vi "UpdateNavxData.vi"(9 "Iterations between saves":i32=10, 10 "Iteration counter":i32, 11 "Datalogging File Refnum in":refnum<k34>) -> (3 "Datalogging File Refnum out":refnum<k34>)   [LabVIEW 2014]
uses:
  Navx_Library/navX-MXP Library/COMMON/TypeDefs/Data TypeDefs/navX Quaternion Data.ctl
  Navx_Library/navX-MXP Library/COMMON/TypeDefs/Data TypeDefs/navX YPRH Data.ctl
  Navx_Library/navX-MXP Library/COMMON/TypeDefs/Data TypeDefs/navX Vector Data.ctl
  Variables/Physical data.vi
  Variables/Default global.vi
  Navx_Library/navX-MXP Library/navX-MXP IMU.lvlib
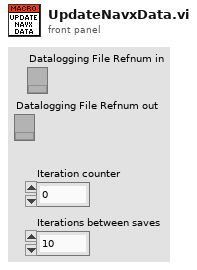
[diagram p1: front panel]
types:
  T1 = typedef "navX-MXP IMU.lvlib/navX Quaternion Data.ctl" = cluster{"W":dbl, "X":dbl, "Y":dbl, "Z":dbl}
  T2 = typedef "navX-MXP IMU.lvlib/navX YPRH Data.ctl" = cluster{"Yaw":dbl, "Pitch":dbl, "Roll":dbl, "Heading":dbl}
  T3 = typedef "navX-MXP IMU.lvlib/navX Vector Data.ctl" = cluster{"X":dbl, "Y":dbl, "Z":dbl}
  T4 = cluster{"Quaternion":T1, "YPRH":T2, "Linear Acceleration":T3, "Valid?":bool}
  T5 = typedef "navX-MXP IMU.lvlib/navX Device TypeDef.ctl" = cluster{"navX Interface Protocol":T6, "navX Interface Protocol TypeDefs":cluster{"SPIDevRef":T7, "I2CDevRef":T10}, "navX System Information":cluster{"Board Information":T12, "Status":T13, "Offsets":T17}, "navX Common Information":cluster{"Update Rate (4Hz-60Hz)":T18, "refnum name":string, "error":errorcluster}}
  T6 = typedef "navX-MXP IMU.lvlib/navX Interface Protocol.ctl" = enum16{"SPI", "I2C"}
  T7 = typedef "WPI_SPIDevRef.ctl" = cluster{"DevStatus":errorcluster, "Handle":i32, "Controller":T8, "SPI Bus":T9}
  T8 = typedef "FPGA_TypedefDigitalModule.ctl" = enum16{"Controller 1"}
  T9 = typedef "spi_bus.ctl" = enum16{"SPI On-Board, CS0", "SPI On-Board, CS1", "SPI On-Board, CS2", "SPI On-Board, CS3", "SPI MXP", "Invalid"}
  T10 = typedef "WPI_I2CDevRef.ctl" = cluster{"DevStatus":errorcluster, "Controller":T8, "Device Address":u8, "Handle":i32, "I2C Bus":T11}
  T11 = typedef "i2c_bus.ctl" = enum16{"I2C On-Board", "I2C MXP", "Invalid"}
  T12 = typedef "navX-MXP IMU.lvlib/navX Board Information.ctl" = cluster{"WhoAmI (50 | 0x32)":u8, "Board Revision":u8, "Firmware Major Version":u8, "Firmware Minor Version":u8}
  T13 = typedef "navX-MXP IMU.lvlib/navX Status Data.ctl" = cluster{"Update Rate Hz":u8, "Accelerometer Full-Scale Range":u8, "Gyro Full-Scale Range":u16, "NAVX_OP_STATUS":T14, "NAVX_CAL_STATUS":T15, "NAVX_SELFTEST_STATUS":u8, "NAVX_SENSOR_STATUS":T16}
  T14 = typedef "navX-MXP IMU.lvlib/navX NAVX_OP_STATUS.ctl" = u8
  T15 = typedef "navX-MXP IMU.lvlib/navX NAVX_CAL_STATUS.ctl" = u8
  T16 = typedef "navX-MXP IMU.lvlib/navX NAVX_SENSOR_STATUS.ctl" = cluster{"MOVING":bool, "YAW_STABLE":bool, "MAG_DISTURBANCE":bool, "ALTITUDE_VALID":bool, "SEALEVEL_PRESS_SET":bool, "FUSED_HEADING_VALID":bool}
  T17 = typedef "navX-MXP IMU.lvlib/navX Offsets Data.ctl" = cluster{"Yaw":dbl, "Quat W":dbl, "Quat X":dbl, "Quat Y":dbl, "Quat Z":dbl}
  T18 = typedef "navX-MXP IMU.lvlib/navX Update Rate.ctl" = u8
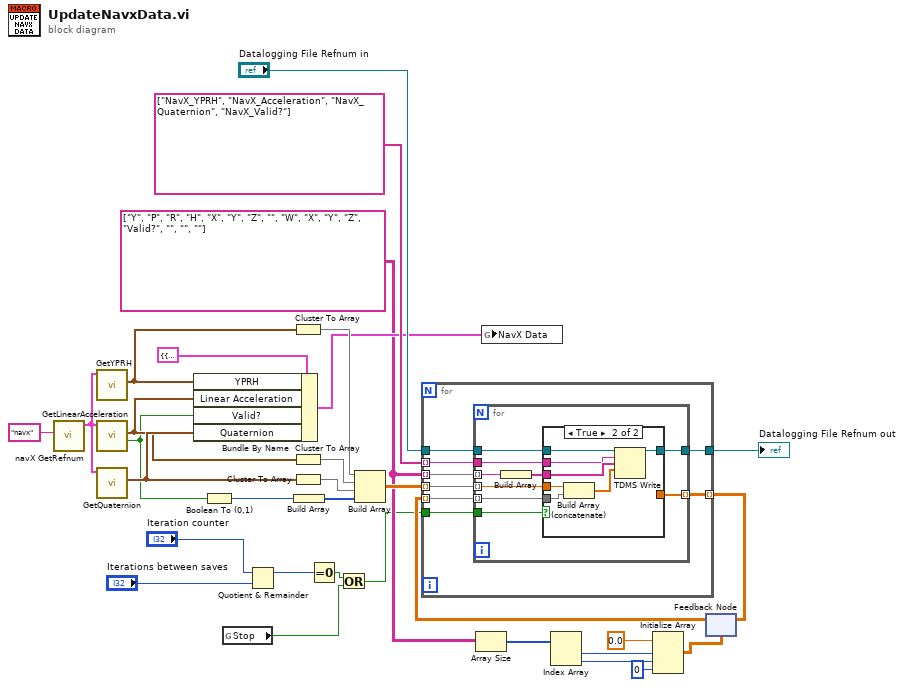
[diagram p0: block diagram]
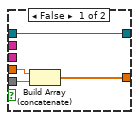
[diagram p2: hidden frame]
diagram:
  w8 = string[][] [["Y", "P", "R", "H"], ["X", "Y", "Z", ""], ["W", "X", "Y", "Z"], ["Valid?", "", "", ""]]
  n1 = call "navX GetRefnum.vi"("refnum name"="navx") -> ("navX Device TypeDef"=w23:T5)  [unwired: 9 in, 1 out]
  n2 = call "GetYPRH.vi"("navX Device TypeDef"=w23) -> ("YPRH"=w25:T2)  [unwired: 8 in, 2 out]
  n3 = call "GetLinearAcceleration.vi"("navX Device TypeDef"=w23) -> ("Valid?"=w21:bool, "Linear Acceleration"=w26:T3)  [unwired: 8 in, 1 out]
  n4 = call "GetQuaternion.vi"("navX Device TypeDef"=w23) -> ("Quaternion"=w27:T1)  [unwired: 8 in, 2 out]
  n5 = Bundle By Name(cluster=T4 {"Quaternion"={"W"=0.0, "X"=0.0, "Y"=0.0, "Z"=0.0}, "YPRH"={"Yaw"=0.0, "Pitch"=0.0, "Roll"=0.0, "Heading"=0.0}, "Linear Acceleration"={"X"=0.0, "Y"=0.0, "Z"=0.0}, "Valid?"=FALSE} ("NavX Data"), "YPRH"=w25, "Linear Acceleration"=w26, "Valid?"=w21, "Quaternion"=w27) -> (w11:T4)
  n6 = Boolean To (0,1)(Boolean=w21) -> (0, 1=w20:i16)
  n7 = global read "Default global.vi" "Stop"() -> (w1:bool)
  n8 = Quotient & Remainder(x="Iteration counter", y="Iterations between saves") -> (x-y*floor(x/y)=w16:i32)  [unwired: 1 out]
  n9 = Cluster To Array(cluster=w25) -> (array=w30:dbl[])
  n10 = Cluster To Array(cluster=w26) -> (array=w29:dbl[])
  n11 = Cluster To Array(cluster=w27) -> (array=w28:dbl[])
  n12 = Build Array(w20) -> (w19:i16[])
  n13 = Equal To 0?(x=w16) -> (x = 0?=w3:bool)
  n14 = Or(x=w3, y=w1) -> (x .or. y?=w2:bool)
  n15 = Build Array(w30, w29, w28, w19) -> (w31:dbl[][])
  n16 = Array Size(array=w8) -> (size(s)=w7:i32[])
  n17 = global write "Physical data.vi" "NavX Data"(w11) -> ()
  n18 = Index Array(array=w7) -> (element #1=w6:i32, element #2=w5:i32)  [unwired: 2 in]
  n19 = Initialize Array(0.0 ("element"), w6, w5, 0 ("dimension size")) -> (w9:dbl[][][])
  n20 = feedback #1(w9) -> (w13:dbl[][][])
  n21 = for {
    tunnel: w8 -> [w39] mode=indexing
    tunnel: w31 -> [w40] mode=indexing
    tunnel: string[] ["NavX_YPRH", "NavX_Acceleration", "NavX_Quaternion", "NavX_Valid?"] -> [w38] mode=indexing
    tunnel: w2 -> [w37]
    tunnel: "Datalogging File Refnum in" -> [w36]
    tunnel: [w35] -> w14 mode=indexing
    tunnel: w13 -> [w34] mode=indexing
    tunnel: [w33] -> w12
    n22 = for {
      tunnel: w40 -> [w48] mode=indexing
      tunnel: w39 -> [w49] mode=indexing
      tunnel: w38 -> [w46]
      tunnel: w37 -> [w47]
      tunnel: w36 -> [w44]
      tunnel: [w43] -> w35 mode=indexing
      tunnel: w34 -> [w42] mode=indexing
      tunnel: [w41] -> w33
      n23 = Build Array(w49) -> (w45:string[])
      n24 = case shown="True" w47 {
        tunnel: w48 -> [w53 w60]
        tunnel: [w52 _] -> w43
        tunnel: w46 -> [_ w56]
        tunnel: w45 -> [_ w57]
        tunnel: w44 -> [w50 w55]
        tunnel: w42 -> [w51 w59]
        tunnel: [w50 w54] -> w41
        frame False {
          n25 = Build Array (concatenate)(w53, w51) -> (w52:dbl[])
        }
        frame True {
          n26 = Build Array (concatenate)(w60, w59) -> (w58:dbl[])
          n27 = TDMS Write(0:w55, 5:w56, 7:w57, 9:w58) -> (4:w54:refnum<k34>)  [unwired: 2 in, 3 out]
        }
      }
    }
  }
  "Datalogging File Refnum out" <- w12
  n28 = feedback-in #1(w14) -> ()
